vi "Telnet Open Connection.vi"(6 "local port":u16, 8 "error in (no error)":errorcluster, 9 "timeout ms (60000)":i32=60000, 10 "remote port (23)":u16=23, 11 "address":string) -> (0 "error out":errorcluster, 3 "telnet connection":T1)   [LabVIEW 2015, in "NI_InternetTK_Core_VIs.lvlib"]
doc: "Opens a Telnet connection using an address and port that you specify."
uses:
  NI_InternetTK_Core_VIs.lvlib
  Telnet Session.ctl
panel:
  in  "<<Timeout>>":bool=TRUE
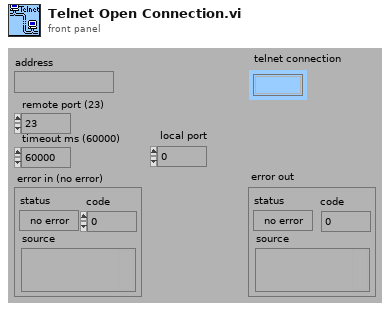
[diagram p1: front panel]
types:
  T1 = typedef "Telnet Session.ctl" = refnum<k1>
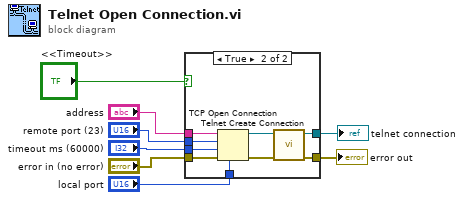
[diagram p0: block diagram]
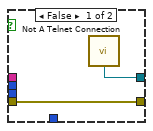
[diagram p2: hidden frame]
diagram:
  n1 = case shown="True" "<<Timeout>>" {
    tunnel: [w9 w19] -> w2
    tunnel: [w10 w18] -> w3
    tunnel: "address" -> [_ w15]
    tunnel: "local port" -> [_ w14]
    tunnel: "timeout ms (60000)" -> [_ w13]
    tunnel: "remote port (23)" -> [_ w12]
    tunnel: "error in (no error)" -> [w9 w11]
    frame False {
      n2 = call "Not A Telnet Connection.vi"() -> ("not a telnet connection"=w10:T1)
    }
    frame True {
      n3 = TCP Open Connection(address=w15, remote port or service name=w12, timeout ms (60000)=w13, local port=w14, error in (no error)=w11) -> (connection ID=w16:refnum<k5>, error out=w17:errorcluster)
      n4 = call "Telnet Create Connection.vi"("error in (no error)"=w17, "TCP connection"=w16) -> ("error out"=w19:errorcluster, "telnet connection"=w18:T1)  [unwired: 8 out]
    }
  }
  "error out" <- w2
  "telnet connection" <- w3
